vi "Read period.vi"(8 "error in (no error)":errorcluster, 11 "Wfm_Amplitude in":refnum<class "Wfm_Amplitude.lvclass">) -> (0 "error out":errorcluster, 1 "high state level":dbl, 2 "amplitude":dbl format="%.2p", 3 "Wfm_Amplitude out":refnum<class "Wfm_Amplitude.lvclass">, 4 "low state level":dbl)   [LabVIEW 2012, in "MyApp.lvlib" / "Wfm_Amplitude.lvclass"]
uses:
  Wfm_Amplitude.lvclass
  Wfm_Amplitude.lvclass/Wfm_Amplitude.ctl
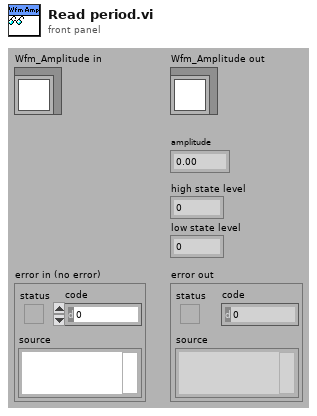
[diagram p1: front panel]
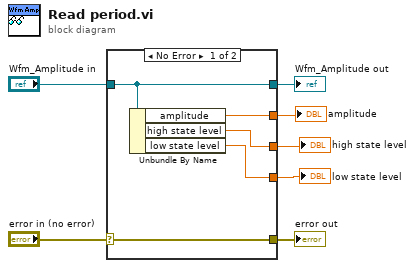
[diagram p0: block diagram]
diagram:
  n1 = case shown="No Error" "error in (no error)" {
    selector: "error in (no error)" -> [w12 w13]
    tunnel: [w12 w13] -> w6
    tunnel: [w11 w14] -> w4
    tunnel: "Wfm_Amplitude in" -> [w11 w14]
    tunnel: [w10 _] -> w3
    tunnel: [w9 _] -> w2
    tunnel: [w8 _] -> w1
    frame No Error {
      n2 = Unbundle By Name(w11) -> ("amplitude"=w10:dbl, "high state level"=w9:dbl, "low state level"=w8:dbl)
    }
    frame Error {
    }
  }
  "error out" <- w6
  "Wfm_Amplitude out" <- w4
  "amplitude" <- w3
  "high state level" <- w2
  "low state level" <- w1
